vi "query.vi"(6 "timeout ms (1000)":i32=1000, 8 "error in (no error)":errorcluster, 10 "Query":string, 11 "TCP in":refnum<k5>) -> (0 "error out":errorcluster, 2 "Return String":string, 3 "TCP out":refnum<k5>)   [LabVIEW 2025, in "Newtons4thEkg.lvlib"]
uses:
  Newtons4thEkg.lvlib
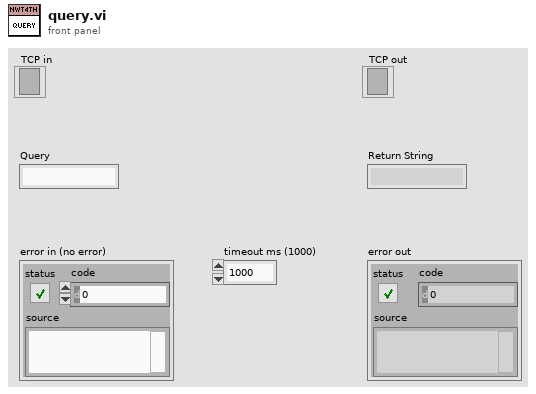
[diagram p1: front panel]
types:
  T1 = enum16{"Standard", "Buffered", "CRLF", "Immediate"}
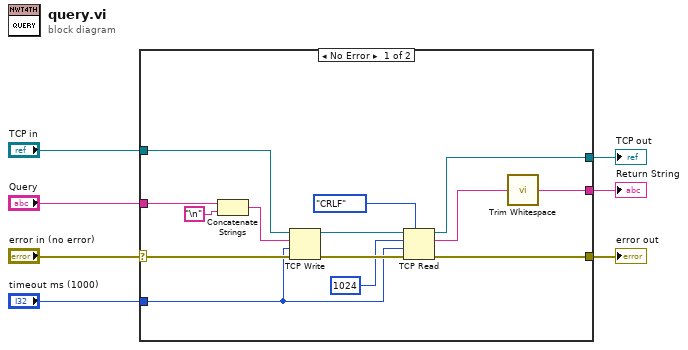
[diagram p0: block diagram]
diagram:
  n1 = case shown="No Error" "error in (no error)" {
    selector: "error in (no error)" -> [w18 w23]
    tunnel: "Query" -> [w21 _]
    tunnel: "TCP in" -> [w17 w22]
    tunnel: "timeout ms (1000)" -> [w9 _]
    tunnel: [w14 w23] -> w3
    tunnel: [w8 _] -> w2
    tunnel: [w12 w22] -> w1
    frame No Error {
      n2 = Concatenate Strings(w21, "\n") -> (w19:string)
      n3 = TCP Write(connection ID=w17, data in=w19, error in (no error)=w18, 9:w9) -> (connection ID out=w16:refnum<k5>, error out=w15:errorcluster)  [unwired: 1 out]
      n4 = TCP Read(connection ID=w16, bytes to read=1024, error in (no error)=w15, 7:T1."CRLF" ("mode (standard)"), 9:w9) -> (connection ID out=w12:refnum<k5>, data out=w13:string, error out=w14:errorcluster)
      n5 = call <vilib>:"Trim Whitespace.vi"("string"=w13) -> ("trimmed string"=w8:string)  [unwired: 1 in]
    }
    frame Error {
    }
  }
  "TCP out" <- w1
  "Return String" <- w2
  "error out" <- w3
